vi "Tacking Helper - Waypoint Array Constructor.vi"(0 "Second Angle":dbl, 1 "Minimum Final Tack Distance (m?)":dbl, 2 "Starting\nArm Length":dbl, 3 "Second\nArm Length":dbl, 5 "Jump Length (m)":dbl, 7 "Starting Angle":dbl, 9 "Distance of each waypoint to boat":dbl[](array[numeric]), 12 "Array Beginning":i32, 13 "Waypoint Array In":T1[](array[typedef]) {"Point Type" items=["Drive", "Round Port", "Round Starboard", "Stay"]}, 14 "Boat Position":T3) -> (4 "Distance to boat":dbl, 6 "Final Index of\nWaypoint Array":i32, 8 "Intermediate \nWaypoint Array out":T1[](array[typedef]) {"Point Type" items=["Drive", "Round Port", "Round Starboard", "Stay"]})   [LabVIEW 2011]
doc: "While the distance to the boat is greater than 1 jump (plus a minimum tack distance allowable we have yet to determine) the while loop will increment again and another two points will be calculated (one jump). The subvi inside of the loop takes the angles and lengths and actually adds the next step to the array.\n\nThe intermediate waypoint array output is the important thing - it stores each waypoint. The 'final index' and 'distance until boat' are used for plotting."
uses:
  2 Typedefs/UTM Location.ctl
  2x3-RIO-OCU Comm/2x3 Typedefs/ocuWaypoint.ctl
  2x3-RIO-OCU Comm/2x3 Typedefs/waypointTypes.ctl
  <vilib>/Analysis/_algsub.llb/Real Vector Norm.vi
  <vilib>/Analysis/NI_AALPro.lvlib
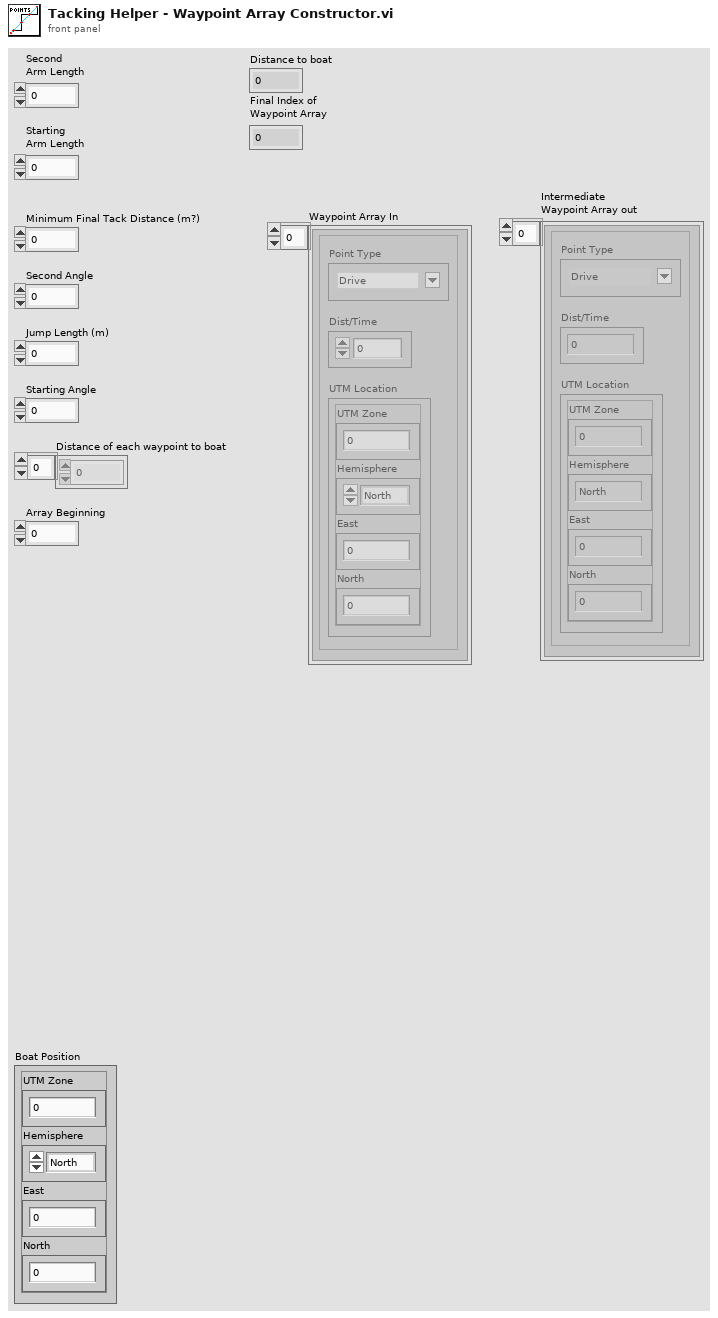
[diagram p1: front panel]
types:
  T1 = typedef "ocuWaypoint.ctl" = cluster{"Point Type":T2, "Dist/Time":dbl, "UTM Location":T3}
  T2 = typedef "waypointTypes.ctl" = u16
  T3 = typedef "UTM Location.ctl" = cluster{"UTM Zone":dbl, "Hemisphere":enum16{"North", "South"}, "East":dbl, "North":dbl}
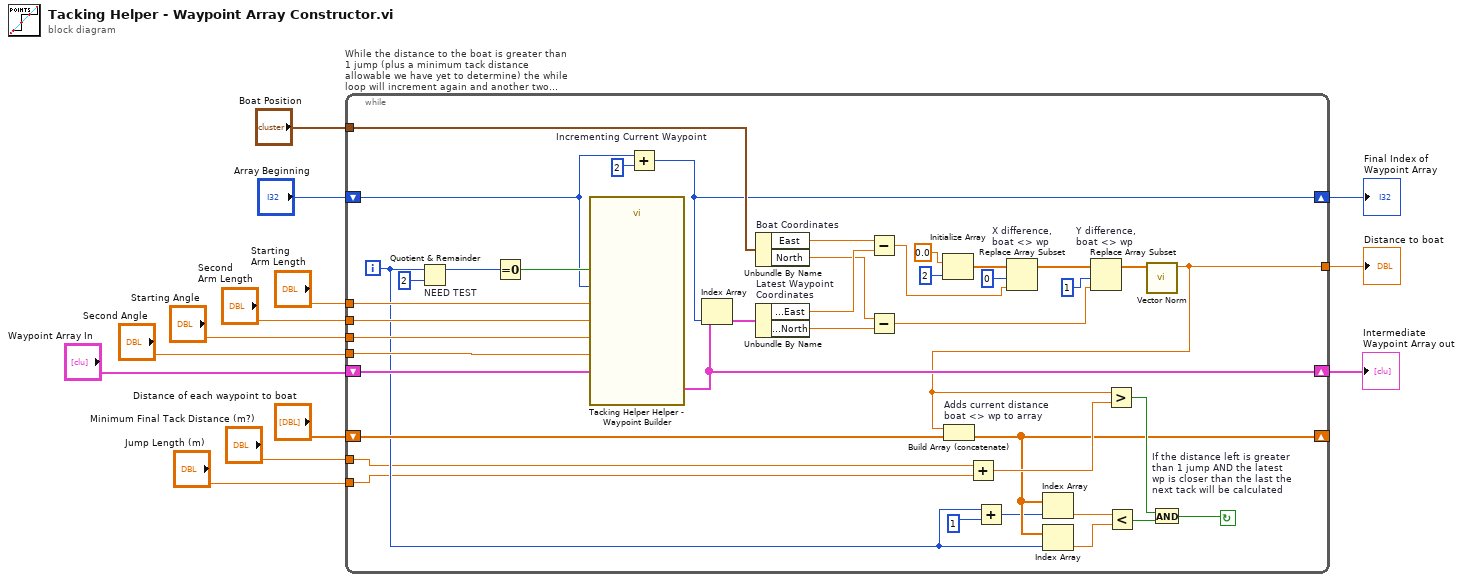
[diagram p0: block diagram]
diagram:
  n1 = while "While the distance to the boat is greater than 1 jump (plus a minimum tack distance allowable we have yet to determine) the while loop will increment again and another two points will be\ncalculated (one jump). The subvi inside of the loop actually takes the angles and lengths and actually adds the next step to the array.." {
    shift-right: [w43] -> w8
    shift-left: "Array Beginning" -> [w50]
    shift-right: [w42] -> w7
    shift-left: "Waypoint Array In" -> [w49]
    tunnel: "Starting\nArm Length" -> [w48]
    tunnel: "Second\nArm Length" -> [w47]
    tunnel: "Starting Angle" -> [w46]
    tunnel: "Second Angle" -> [w45]
    tunnel: "Boat Position" -> [w44]
    tunnel: "Jump Length (m)" -> [w15]
    shift-right: [w22] -> _
    shift-left: "Distance of each waypoint to boat" -> [w24]
    tunnel: [w14] -> w9
    tunnel: "Minimum Final Tack Distance (m?)" -> [w16]
    i -> [w19]
    stop <- w25 continue-if-true
    n2 = Quotient & Remainder "NEED TEST"(x=w19, y=2) -> (x-y*floor(x/y)=w51:i32)  [unwired: 1 out]
    n3 = Equal To 0?(x=w51) -> (x = 0?=w52:bool)
    n4 = call "Tacking Helper Helper - Waypoint Builder.vi"("Second Arm Length"=w47, "Current Waypoint\nBeing Adjusted"=w50, "Starting Arm Length"=w48, "Waypoint\nArray In"=w49, "Second Angle"=w45, "Is the jump even or odd?\nEven jumps use the starting\nangle first, odd the secondary"=w52, "Starting Angle"=w46) -> ("Waypoint \nArray Out"=w42:T1[])  [unwired: 4 in]
    n5 = Add "Incrementing Current Waypoint"(x=w50, y=2) -> (x+y=w43:i32)
    n6 = Index Array(array=w42, index=w43) -> (element=w41:T1)
    n7 = Unbundle By Name "Boat Coordinates"(w44) -> ("East"=w40:dbl, "North"=w38:dbl)
    n8 = Unbundle By Name "Latest Waypoint\nCoordinates"(w41) -> ("UTM Location.East"=w39:dbl, "UTM Location.North"=w37:dbl)
    n9 = Subtract(x=w40, y=w39) -> (x-y=w32:dbl)
    n10 = Subtract(x=w38, y=w37) -> (x-y=w29:dbl)
    n11 = Initialize Array(0.0 ("element"), 2 ("dimension size")) -> (w34:dbl[])
    n12 = Add(x=w16, y=w15) -> (x+y=w27:dbl)
    n13 = Add(x=w19, y=1) -> (x+y=w17:i32)
    n14 = Replace Array Subset "X difference,\nboat <> wp"(array=w34, new element=w32, index=0) -> (w30:dbl[])
    n15 = Replace Array Subset "Y difference,\nboat <> wp"(array=w30, new element=w29, index=1) -> (w28:dbl[])
    n16 = call-poly <vilib>:"Vector Norm.vi"("Input Vector"=w28) -> ("norm"=w14:dbl)  [unwired: 9 in, 1 out]
    n17 = Build Array (concatenate) "Adds current distance\nboat <> wp to array"(w14, w24) -> (w22:dbl[])
    n18 = Index Array(array=w22, index=w17) -> (element=w23:dbl)
    n19 = Index Array(array=w22, index=w19) -> (element=w21:dbl)
    n20 = Greater?(x=w14, y=w27) -> (0:w26:bool)
    n21 = Less?(x=w23, y=w21) -> (x < y?=w20:bool)
    n22 = And "If the distance left is greater\nthan 1 jump AND the latest\nwp is closer than the last the\nnext tack will be calculated"(x=w26, y=w20) -> (x .and. y?=w25:bool)
  }
  "Distance to boat" <- w9
  "Final Index of\nWaypoint Array" <- w8
  "Intermediate \nWaypoint Array out" <- w7
